vi "Prefilter_LP.vi"(8 "error in (no error)":errorcluster, 9 "ON?":bool, 10 "high cutoff freq [Hz]":dbl=0.45, 11 "Instrument.DAQ":refnum<class "Instrument.DAQ.lvclass">) -> (0 "error out":errorcluster, 3 "Instrument.DAQ out":refnum<class "Instrument.DAQ.lvclass">)   [LabVIEW 2019, in "Instrument.DAQ.lvclass"]
uses:
  Instrument.DAQ.lvclass
  Instrument.DAQ.lvclass/Instrument.DAQ.ctl
  <vilib>/addons/Digital Filter Design/Process.llb/DFD Filtering (Wfm NChan).vi
  <vilib>/addons/Digital Filter Design/NI_DigFilterLicensed.lvlib
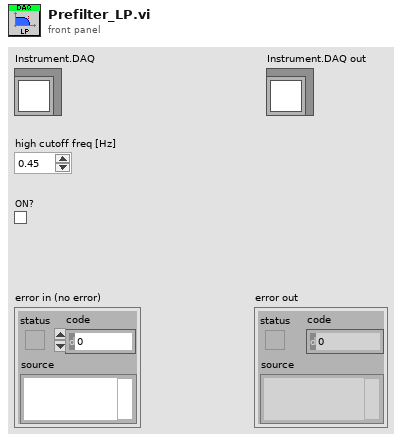
[diagram p1: front panel]
types:
  T1 = enum16{"Lowpass", "Highpass", "Bandpass", "Bandstop"}
  T2 = typedef "Instrument.DAQ.lvclass/PublicEvents--DAQ.getWaveforms.ctl" = cluster{"AO":waveform(dbl)[], "AI":waveform(dbl)[], "RefX":waveform(dbl)[], "RefY":waveform(dbl)[]}
  T3 = typedef "NI_DigFilterLicensed.lvlib/DFD Filter Obj.ctl" = cluster{"mSRate_Fs":dbl, "mSRate_Version":string, "mSRate_Comments":string, "mSRate_OrgCoef":T4, "mSRate_CurCoef":T4, "mSRate_Quantized?":bool, "mSRate_QCoef":T4, "mSRate_QSettings":T6[], "mSRate_Order":i32, "mSRate_Scaling":cluster{"mSRate_ScaleByPowerOf2?":bool, "mSRate_ScaleType":T8}}
  T4 = typedef "NI_DigFilterLicensed.lvlib/DFD Filter Coef.ctl" = cluster{"type":T5, "gain":dbl, "coef a (k)":dbl[], "coef b (v)":dbl[]}
  T5 = typedef "NI_DigFilterLicensed.lvlib/DFD Filter Structure Type Selector.ctl" = enum16{"Undefined", "FIR Direct Form", "FIR Direct Form Transposed", "FIR Symmetric", "FIR Antisymmetric", "IIR Direct Form I", "IIR Direct Form I Transposed", "IIR Direct Form II", "IIR Direct Form II Transposed", "IIR Cascaded Second Order Sections Form I", "IIR Cascaded Second Order Sections Form I Transposed", "IIR Cascaded Second Order Sections Form II", "IIR Cascaded Second Order Sections Form II Transposed", "Lattice Allpass (basic sections)", "Lattice Allpass (one multiplier sections)", "Lattice Allpass (normalized sections)", "Lattice AR (basic sections)", "Lattice AR (one multiplier sections)", "Lattice AR (normalized sections)", "Lattice MA (minimum phase)", "Lattice MA (maximum phase)", "Lattice ARMA (basic sections)", "Lattice ARMA (one multiplier sections)", "Lattice ARMA (normalized sections)"}
  T6 = typedef "NI_DigFilterLicensed.lvlib/dfd_Internal Quantization Settings.ctl" = cluster{"source":T7, "wl":i16, "iwl":i16, "overflow mode":enum16{"Saturation", "Wrap"}, "rounding mode":enum16{"Nearest", "Truncation"}, "signed?":bool}
  T7 = typedef "NI_DigFilterLicensed.lvlib/dfd_Internal Quantization Srcs.ctl" = u16
  T8 = typedef "NI_DigFilterLicensed.lvlib/DFD Coef Norm Type.ctl" = enum16{"No Norm", "Time Domain 1-Norm", "Time Domain 2-Norm", "Time Domain Inf-Norm"}
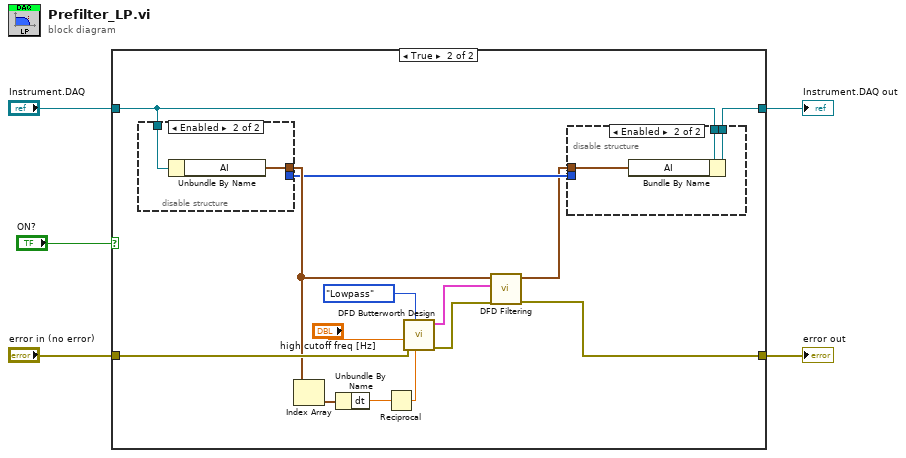
[diagram p0: block diagram]
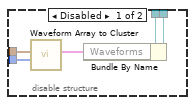
[diagram p3: hidden frame]
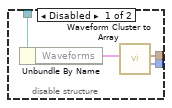
[diagram p4: hidden frame]
diagram:
  n1 = case shown="True" "ON?" {
    tunnel: "error in (no error)" -> [w6 w15]
    tunnel: [w6 w13] -> w4
    tunnel: "Instrument.DAQ" -> [w7 w11]
    tunnel: [w7 w10] -> w2
    frame False {
    }
    frame True {
      n2 = disable-structure shown="Enabled" {
        disable-tunnel: [w33 w34] -> w12
        disable-tunnel: w11 -> [w32 w35]
        disable-tunnel: [w30 _] -> w9
        frame Disabled {
          n3 = Unbundle By Name(w32) -> ("Waveforms"=w31:T2)
          n4 = call "Waveform Cluster to Array.vi"("Waveform Cluster"=w31) -> ("Lengths"=w30:i32[], "Concatenated Waveforms"=w33:waveform(dbl)[])  [unwired: 9 in]
        }
        frame Enabled {
          n5 = Unbundle By Name(w35) -> ("AI"=w34:waveform(dbl)[])
        }
      }
      n6 = Index Array(array=w12) -> (element=w20:waveform(dbl))  [unwired: 1 in]
      n7 = Unbundle By Name(w20) -> ("dt"=w21:dbl)
      n8 = Reciprocal(x=w21) -> (1/x=w19:dbl)
      n9 = call <vilib>:"DFD Butterworth Design.vi"("fs [Hz]"=w19, "filter type"=T1."Lowpass", "error in (no error)"=w15, "low cutoff freq [Hz]"="high cutoff freq [Hz]") -> ("error out"=w14:errorcluster, "filter out"=w18:T3)  [unwired: 6 in]
      n10 = call-poly <vilib>:"DFD Filtering.vi"("error in (no error)"=w14, "filter"=w18, "signal in"=w12) -> ("error out"=w13:errorcluster, "signal out"=w8:waveform(dbl)[])  [unwired: 7 in]
      n11 = disable-structure shown="Enabled" {
        disable-tunnel: w11 -> [w26 w29]
        disable-tunnel: [w25 w28] -> w10
        disable-tunnel: w9 -> [w23 _]
        disable-tunnel: w8 -> [w22 w27]
        frame Disabled {
          n12 = call "Waveform Array to Cluster.vi"("Lengths"=w23, "Concatenated Waveforms"=w22) -> ("Waveform Cluster"=w24:T2)  [unwired: 9 in]
          n13 = Bundle By Name(cluster=w26, "Waveforms"=w24) -> (w25:refnum<class "Instrument.DAQ.lvclass">)
        }
        frame Enabled {
          n14 = Bundle By Name(cluster=w29, "AI"=w27) -> (w28:refnum<class "Instrument.DAQ.lvclass">)
        }
      }
    }
  }
  "error out" <- w4
  "Instrument.DAQ out" <- w2
